vi "Close device.vi"(1 "error in (no error)":errorcluster, 2 "handle":u32) -> (0 "error out":errorcluster)   [LabVIEW 2013]
uses:
  lib/FTCSPI.dll
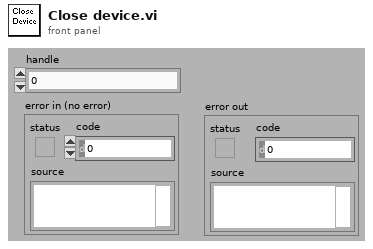
[diagram p1: front panel]
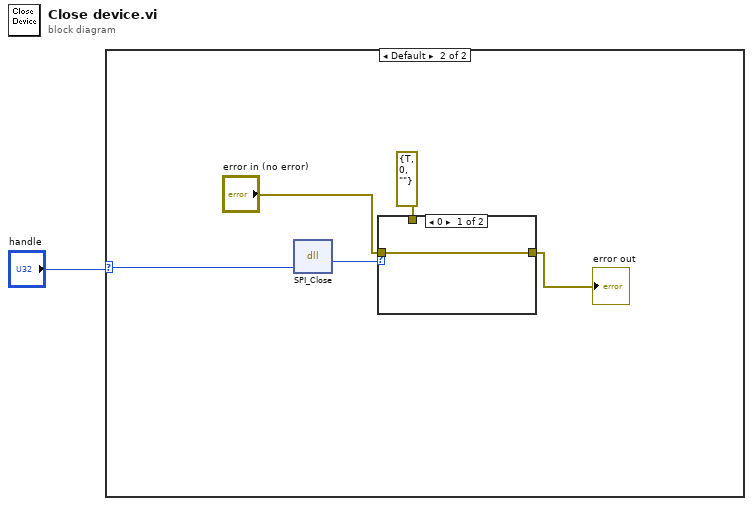
[diagram p0: block diagram]
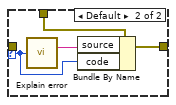
[diagram p3: hidden frame]
diagram:
  n1 = case shown="Default" "handle" {
    selector: "handle" -> [_ w2]
    frame 0 {
    }
    frame Default {
      n2 = dll-call lib="C:/Users/SuperUser/Documents/HiSparc/hisparcdaq/FPGA/lib/FTCSPI.dll" fn="SPI_Close"("handle"=w2) -> ("result"=w5:u32)  [unwired: 4 in, 2 out]
      n3 = case shown="0" w5 {
        selector: w5 -> [_ w8]
        tunnel: "error in (no error)" -> [w7 _]
        tunnel: [w7 w10] -> w6
        tunnel: errorcluster {"status"=TRUE, "code"=0, "source"=""} ("error out") -> [_ w11]
        frame 0 {
        }
        frame Default {
          n4 = call "Explain error.vi"("error"=w8) -> ("error string"=w9:string)
          n5 = Bundle By Name(cluster=w11, "source"=w9, "code"=w8) -> (w10:errorcluster)
        }
      }
      "error out" <- w6
    }
  }
